vi "SSS_RX_GENERATE(SubVI).vi"(0 "OSC_Frequency(Hz)":dbl=430000.0 format="%#_6p", 1 "OSC_Pulse length(sec)":dbl=0.0004 format="%#_6p", 2 "TXEN_Pulse length(sec)":dbl=0.0004 format="%#_6p", 5 "STC_Pulse length(sec)":dbl=1.0 format="%#_6p", 7 "STC_STEP":enum16{"0", "1", "2", "3", "4", "5", "6", "7"}(ring), 9 "STC_Sampling Frequency(Hz)":dbl=192000.0 format="%0.2f", 12 "GAIN_Pulse length(sec)":dbl=1.0 format="%#_6p") -> (3 "Sampling Rate(EN, OSC)":dbl format="%#_3p", 4 "TXEN":waveform(dbl)(graph), 6 "OSC":waveform(dbl)(graph), 8 "STC":waveform(dbl)(graph), 10 "x*y":dbl, 14 "GAIN":waveform(dbl)(graph))   [LabVIEW 2017]
uses:
  <vilib>/Analysis/NI_AALBase.lvlib
panel:
  in  "GAIN_Voltage(V)":dbl
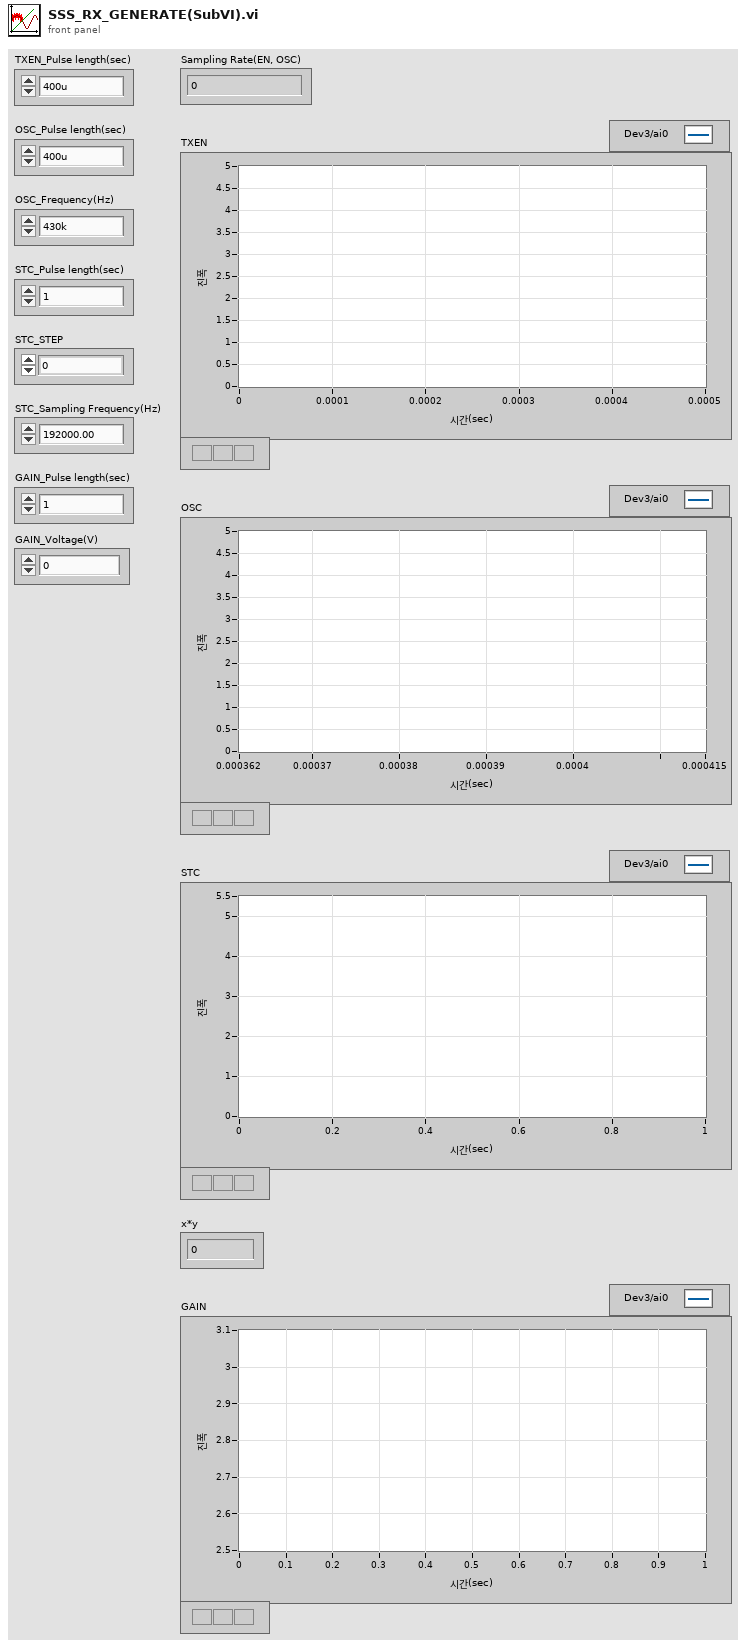
[diagram p1: front panel]
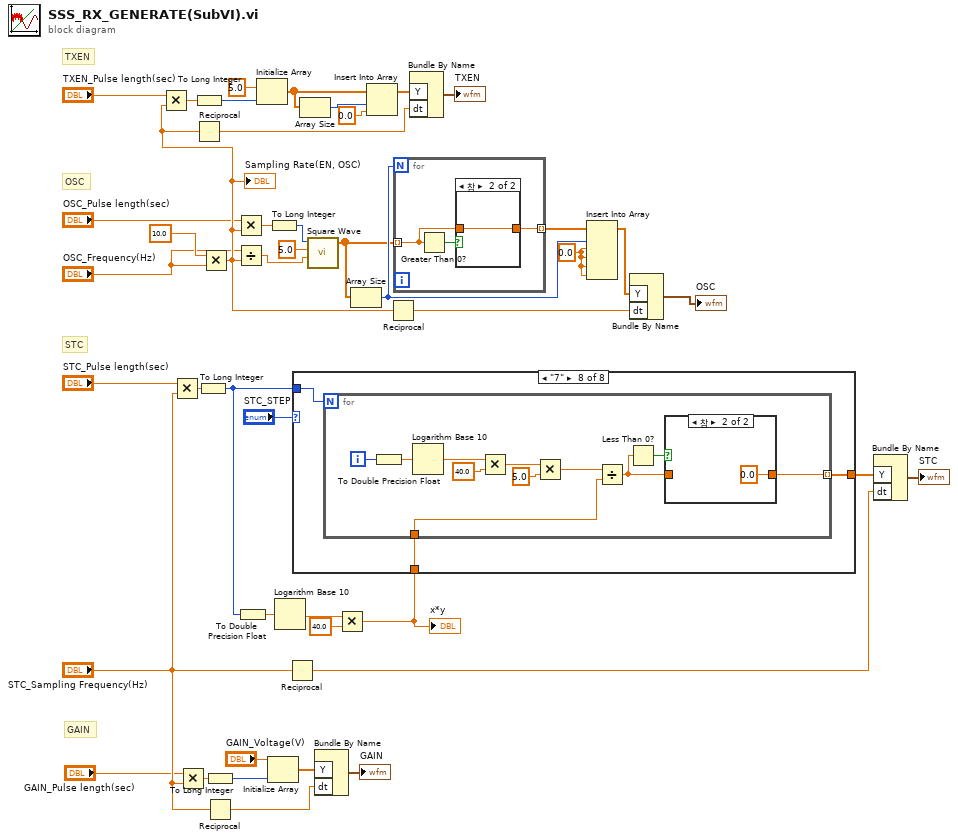
[diagram p0: block diagram]
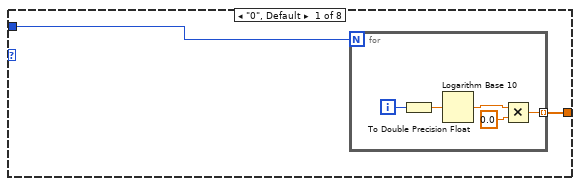
[diagram p2: hidden frame]
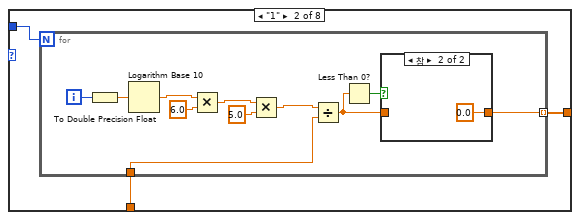
[diagram p3: hidden frame]
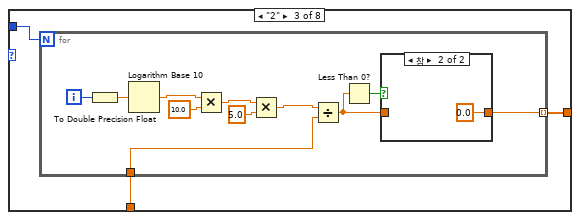
[diagram p5: hidden frame]
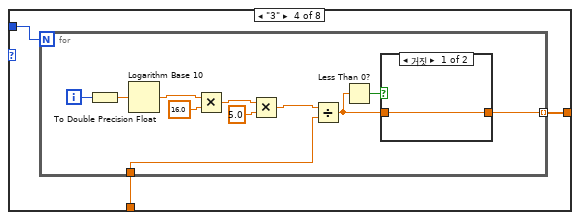
[diagram p7: hidden frame]
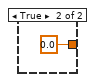
[diagram p8: hidden frame]
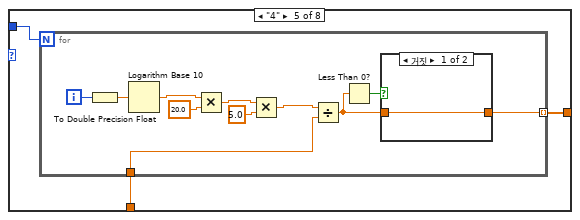
[diagram p9: hidden frame]
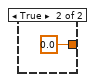
[diagram p10: hidden frame]
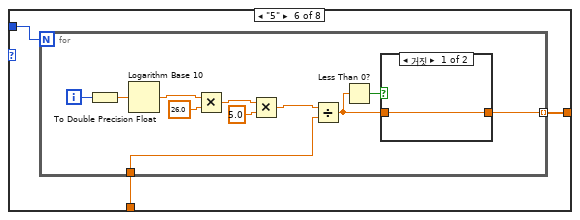
[diagram p11: hidden frame]
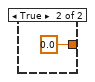
[diagram p12: hidden frame]
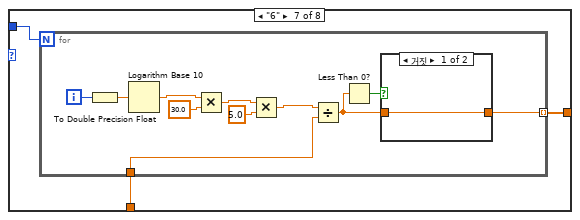
[diagram p13: hidden frame]
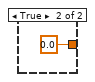
[diagram p14: hidden frame]
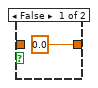
[diagram p16: hidden frame]
diagram:
  w20 = 0.0 ("새 원소/부분배열")
  # "GAIN"
  # "STC"
  # "OSC"
  # "TXEN"
  n1 = Multiply(x="STC_Pulse length(sec)", y="STC_Sampling Frequency(Hz)") -> (x*y=w27:dbl)
  n2 = Multiply(x="GAIN_Pulse length(sec)", y="STC_Sampling Frequency(Hz)") -> (x*y=w34:dbl)
  n3 = To Long Integer(number=w27) -> (32bit integer=w41:i32)
  n4 = Multiply(x=10.0, y="OSC_Frequency(Hz)") -> (x*y=w32:dbl)
  "Sampling Rate(EN, OSC)" <- w32
  n5 = Multiply(x="TXEN_Pulse length(sec)", y=w32) -> (x*y=w3:dbl)
  n6 = To Long Integer(number=w3) -> (32bit integer=w4:i32)
  n7 = Reciprocal(x=w32) -> (1/x=w6:dbl)
  n8 = To Long Integer(number=w34) -> (32bit integer=w35:i32)
  n9 = Reciprocal(x="STC_Sampling Frequency(Hz)") -> (1/x=w36:dbl)
  n10 = Multiply(x="OSC_Pulse length(sec)", y=w32) -> (x*y=w13:dbl)
  n11 = Divide(x="OSC_Frequency(Hz)", y=w32) -> (x/y=w16:dbl)
  n12 = To Double Precision Float(number=w41) -> (double precision float=w40:dbl)
  n13 = Initialize Array(5.0 ("원소"), w4) -> (w8:dbl[])
  n14 = Initialize Array("GAIN_Voltage(V)", w35) -> (w39:dbl[])
  n15 = To Long Integer(number=w13) -> (32bit integer=w14:i32)
  n16 = Logarithm Base 10(1:w40) -> (0:w43:dbl)
  n17 = Reciprocal(x="STC_Sampling Frequency(Hz)") -> (1/x=w28:dbl)
  n18 = Array Size(array=w8) -> (size(s)=w9:i32)
  n19 = call <vilib>:"Square Wave.vi"("samples"=w14, "amplitude"=5.0, "frequency"=w16) -> ("square wave"=w17:dbl[])  [unwired: 3 in, 2 out]
  n20 = Bundle By Name("Y"=w39, "dt"=w36) -> (→"GAIN":waveform(dbl))  [unwired: 1 in]
  n21 = Multiply(x=w43, y=40.0) -> (x*y=w44:dbl)
  "x*y" <- w44
  n22 = case shown="\"7\"" "STC_STEP" {
    tunnel: w41 -> [w46 w54 w70 w86 w102 w118 w134 w150]
    tunnel: [w45 w53 w69 w85 w101 w117 w133 w149] -> w30
    tunnel: w44 -> [_ w52 w68 w84 w100 w116 w132 w148]
    frame "0", Default {
      n23 = for {
        N: w46 -> [_]
        tunnel: [w47] -> w45 mode=indexing
        i -> [w50]
        n24 = To Double Precision Float(number=w50) -> (double precision float=w51:dbl)
        n25 = Logarithm Base 10(1:w51) -> (0:w49:dbl)
        n26 = Multiply(x=w49, y=0.0) -> (x*y=w47:dbl)
      }
    }
    frame "1" {
      n27 = for {
        N: w54 -> [_]
        tunnel: [w57] -> w53 mode=indexing
        tunnel: w52 -> [w55]
        i -> [w64]
        n28 = To Double Precision Float(number=w64) -> (double precision float=w65:dbl)
        n29 = Logarithm Base 10(1:w65) -> (0:w63:dbl)
        n30 = Multiply(x=w63, y=6.0) -> (x*y=w59:dbl)
        n31 = Multiply(x=w59, y=5.0) -> (x*y=w60:dbl)
        n32 = Divide(x=w60, y=w55) -> (x/y=w56:dbl)
        n33 = Less Than 0?(x=w56) -> (x < 0?=w58:bool)
        n34 = case shown="참" w58 {
          tunnel: [w66 0.0] -> w57
          tunnel: w56 -> [w66 _]
          frame False {
          }
          frame True {
          }
        }
      }
    }
    frame "2" {
      n35 = for {
        N: w70 -> [_]
        tunnel: [w72] -> w69 mode=indexing
        tunnel: w68 -> [w71]
        i -> [w80]
        n36 = To Double Precision Float(number=w80) -> (double precision float=w81:dbl)
        n37 = Logarithm Base 10(1:w81) -> (0:w79:dbl)
        n38 = Multiply(x=w79, y=10.0) -> (x*y=w75:dbl)
        n39 = Multiply(x=w75, y=5.0) -> (x*y=w76:dbl)
        n40 = Divide(x=w76, y=w71) -> (x/y=w73:dbl)
        n41 = Less Than 0?(x=w73) -> (x < 0?=w74:bool)
        n42 = case shown="참" w74 {
          tunnel: [w82 0.0] -> w72
          tunnel: w73 -> [w82 _]
          frame False {
          }
          frame True {
          }
        }
      }
    }
    frame "3" {
      n43 = for {
        N: w86 -> [_]
        tunnel: [w88] -> w85 mode=indexing
        tunnel: w84 -> [w87]
        i -> [w96]
        n44 = To Double Precision Float(number=w96) -> (double precision float=w97:dbl)
        n45 = Logarithm Base 10(1:w97) -> (0:w95:dbl)
        n46 = Multiply(x=w95, y=16.0) -> (x*y=w91:dbl)
        n47 = Multiply(x=w91, y=5.0) -> (x*y=w92:dbl)
        n48 = Divide(x=w92, y=w87) -> (x/y=w89:dbl)
        n49 = Less Than 0?(x=w89) -> (x < 0?=w90:bool)
        n50 = case shown="거짓" w90 {
          tunnel: [w98 0.0] -> w88
          tunnel: w89 -> [w98 _]
          frame False {
          }
          frame True {
          }
        }
      }
    }
    frame "4" {
      n51 = for {
        N: w102 -> [_]
        tunnel: [w104] -> w101 mode=indexing
        tunnel: w100 -> [w103]
        i -> [w112]
        n52 = To Double Precision Float(number=w112) -> (double precision float=w113:dbl)
        n53 = Logarithm Base 10(1:w113) -> (0:w111:dbl)
        n54 = Multiply(x=w111, y=20.0) -> (x*y=w107:dbl)
        n55 = Multiply(x=w107, y=5.0) -> (x*y=w108:dbl)
        n56 = Divide(x=w108, y=w103) -> (x/y=w105:dbl)
        n57 = Less Than 0?(x=w105) -> (x < 0?=w106:bool)
        n58 = case shown="거짓" w106 {
          tunnel: [w114 0.0] -> w104
          tunnel: w105 -> [w114 _]
          frame False {
          }
          frame True {
          }
        }
      }
    }
    frame "5" {
      n59 = for {
        N: w118 -> [_]
        tunnel: [w120] -> w117 mode=indexing
        tunnel: w116 -> [w119]
        i -> [w128]
        n60 = To Double Precision Float(number=w128) -> (double precision float=w129:dbl)
        n61 = Logarithm Base 10(1:w129) -> (0:w127:dbl)
        n62 = Multiply(x=w127, y=26.0) -> (x*y=w123:dbl)
        n63 = Multiply(x=w123, y=5.0) -> (x*y=w124:dbl)
        n64 = Divide(x=w124, y=w119) -> (x/y=w121:dbl)
        n65 = Less Than 0?(x=w121) -> (x < 0?=w122:bool)
        n66 = case shown="거짓" w122 {
          tunnel: [w130 0.0] -> w120
          tunnel: w121 -> [w130 _]
          frame False {
          }
          frame True {
          }
        }
      }
    }
    frame "6" {
      n67 = for {
        N: w134 -> [_]
        tunnel: [w136] -> w133 mode=indexing
        tunnel: w132 -> [w135]
        i -> [w144]
        n68 = To Double Precision Float(number=w144) -> (double precision float=w145:dbl)
        n69 = Logarithm Base 10(1:w145) -> (0:w143:dbl)
        n70 = Multiply(x=w143, y=30.0) -> (x*y=w139:dbl)
        n71 = Multiply(x=w139, y=5.0) -> (x*y=w140:dbl)
        n72 = Divide(x=w140, y=w135) -> (x/y=w137:dbl)
        n73 = Less Than 0?(x=w137) -> (x < 0?=w138:bool)
        n74 = case shown="거짓" w138 {
          tunnel: [w146 0.0] -> w136
          tunnel: w137 -> [w146 _]
          frame False {
          }
          frame True {
          }
        }
      }
    }
    frame "7" {
      n75 = for {
        N: w150 -> [_]
        tunnel: [w152] -> w149 mode=indexing
        tunnel: w148 -> [w151]
        i -> [w160]
        n76 = To Double Precision Float(number=w160) -> (double precision float=w161:dbl)
        n77 = Logarithm Base 10(1:w161) -> (0:w159:dbl)
        n78 = Multiply(x=w159, y=40.0) -> (x*y=w157:dbl)
        n79 = Multiply(x=w157, y=5.0) -> (x*y=w155:dbl)
        n80 = Divide(x=w155, y=w151) -> (x/y=w153:dbl)
        n81 = Less Than 0?(x=w153) -> (x < 0?=w154:bool)
        n82 = case shown="참" w154 {
          tunnel: [w162 0.0] -> w152
          tunnel: w153 -> [w162 _]
          frame False {
          }
          frame True {
          }
        }
      }
    }
  }
  n83 = Array Size(array=w17) -> (size(s)=w19:i32)
  n84 = Insert Into Array(array=w8, index=w9, new element=0.0 ("새 원소/부분배열")) -> (w11:dbl[])
  n85 = Reciprocal(x=w32) -> (1/x=w22:dbl)
  n86 = for {
    N: w19 -> [_]
    tunnel: w17 -> [w165] mode=indexing
    tunnel: [w164] -> w18 mode=indexing
    n87 = Greater Than 0?(x=w165) -> (x > 0?=w166:bool)
    n88 = case shown="참" w166 {
      tunnel: w165 -> [_ w168]
      tunnel: [0.0 w168] -> w164
      frame False {
      }
      frame True {
      }
    }
  }
  n89 = Bundle By Name("Y"=w11, "dt"=w6) -> (→"TXEN":waveform(dbl))  [unwired: 1 in]
  n90 = Insert Into Array(array=w18, index=w19, new element #1=w20, new element #2=w20, new element #3=w20, new element #4=w20) -> (w21:dbl[])
  n91 = Bundle By Name("Y"=w21, "dt"=w22) -> (→"OSC":waveform(dbl))  [unwired: 1 in]
  n92 = Bundle By Name("Y"=w30, "dt"=w28) -> (→"STC":waveform(dbl))  [unwired: 1 in]
